vi "Show_Error.vi"(8 "error in (no error)":errorcluster, 11 "DAQmxTaksContainer_General in":refnum<class "DAQmxTaksContainer_General.lvclass">) -> (0 "error out":errorcluster, 3 "DAQmxTaksContainer_General out":refnum<class "DAQmxTaksContainer_General.lvclass">)   [LabVIEW 2018, in "DAQmxTaksContainer_General.lvclass"]
uses:
  DAQmxTaksContainer_General.lvclass
  C:/Users/Sergey Denisov/Documents/REPS/TRANCON/Classes/GeneralFunctionality/GeneralFunctionality.lvclass
  GeneralFunctionality/GeneralFunctionality.lvclass/GeneralFunctionality.ctl
  GeneralFunctionality/GeneralFunctionality.lvclass
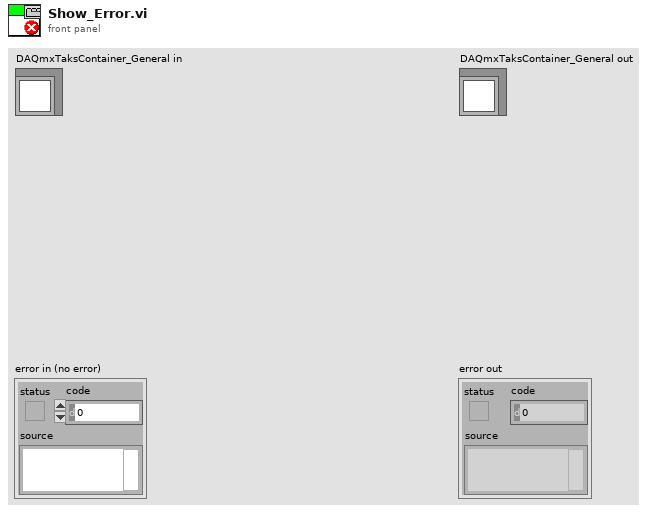
[diagram p1: front panel]
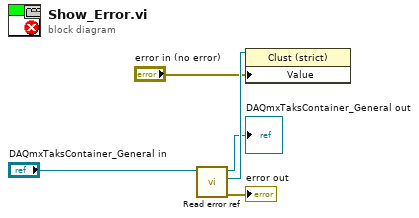
[diagram p0: block diagram]
diagram:
  n1 = call "Read error ref.vi"("GeneralFunctionality in"="DAQmxTaksContainer_General in") -> ("error out"=→"error out":errorcluster, "error"=w5:refnum<vi>, "GeneralFunctionality out"=→"DAQmxTaksContainer_General out":refnum<class "DAQmxTaksContainer_General.lvclass">)  [unwired: 8 in]
  n2 = property class="Clust (strict)"(reference=w5, "Value"="error in (no error)") -> ()  [unwired: 1 in, 2 out]
